vi "Write FilePath.vi"(8 "error in (no error)":errorcluster, 10 "FilePath":path=path "C:/TrigBoxSettings/Settings.ini", 11 "GenericFileClass in":refnum<class "GenericFileClass.lvclass">) -> (0 "error out":errorcluster, 3 "GenericFileClass out":refnum<class "GenericFileClass.lvclass">)   [LabVIEW 2013, in "GenericFileClass.lvclass"]
uses:
  GenericFileClass.lvclass
  GenericFileClass.lvclass/GenericFileClass.ctl
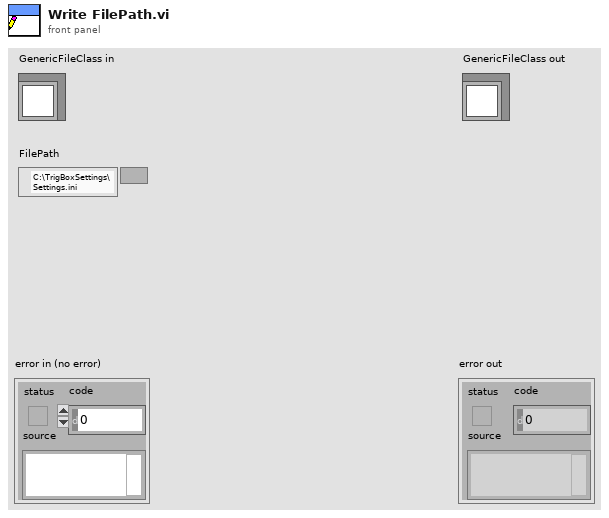
[diagram p1: front panel]
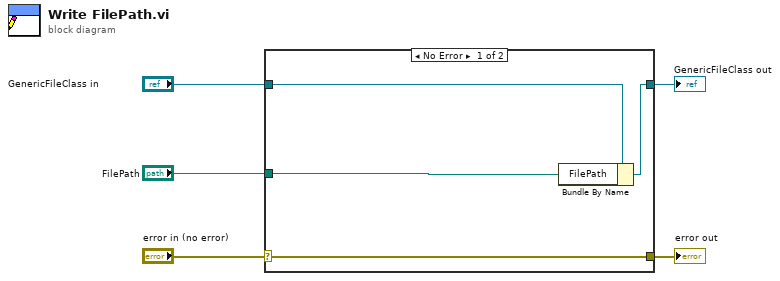
[diagram p0: block diagram]
diagram:
  n1 = case shown="No Error" "error in (no error)" {
    selector: "error in (no error)" -> [w9 w10]
    tunnel: [w9 w10] -> w4
    tunnel: [w7 w11] -> w2
    tunnel: "GenericFileClass in" -> [w8 w11]
    tunnel: "FilePath" -> [w6 _]
    frame No Error {
      n2 = Bundle By Name(cluster=w8, "FilePath"=w6) -> (w7:refnum<class "GenericFileClass.lvclass">)
    }
    frame Error {
    }
  }
  "error out" <- w4
  "GenericFileClass out" <- w2
